vi "Target.vi"() -> ()   [LabVIEW 2019]
uses:
  <vilib>/Platform/TimedLoop/XDataNode/timing_clust.ctl
  <vilib>/Platform/TimedLoop/XDataNode/nitl_modes.ctl
  <vilib>/Platform/TimedLoop/XDataNode/wakeup.ctl
  <vilib>/rvi/Emulation/niFpgaSctlEmulationGetInTimedLoop.vi
  <vilib>/rvi/Emulation/niFpgaEmulationReportErrorSimple.vi
  <vilib>/rvi/Emulation/niFpgaGetClockAttributes.vi
  <vilib>/rvi/Emulation/niFpgaCriticalErrorInLSC.vi
  <vilib>/rvi/DataTransferAndStorage/Container/Common/niFpgaContainerExecOnDevCompGetState.vi
  <vilib>/rvi/errors/niFpgaSetErrorForExecOnDevCompSimple.vi
  <vilib>/rvi/eio/common/nirviEmuReportErrorAndStop.vi
  <vilib>/rvi/interface/RandomDataEmulation/nirviRandomDataAcquireLock.vi
  <vilib>/rvi/interface/RandomDataEmulation/nirviRandomDataQueueStore.vi
  <vilib>/rvi/interface/RandomDataEmulation/nirviRandomDataReleaseLock.vi
  <vilib>/rvi/interface/RandomDataEmulation/nirviFPGAContextMergeError.vi
  <vilib>/rvi/interface/RandomDataEmulation/nirviRandomDataCheckExitLoopConditions.vi
  <vilib>/express/rvi/timingcommon/nirviCommon.vi
  <vilib>/rvi/interface/RandomDataEmulation/niFpgaRandomDataHandleErrors.vi
  <vilib>/rvi/Emulation/niFpgaEmulationIsFPGAContextNoSignature.vi
  <vilib>/rvi/DataTransferAndStorage/Container/Common/niFpgaContainerGetUniqueNameForEmu.vi
  <vilib>/rvi/FIFO/Fifo_Resource/nirvififoEmulationSetSize.vi
  <vilib>/rvi/FIFO/Fifo_Resource/nirviFifoEmulationQueueMgr.vi
  <instcachedir>/0/nirviFifoEmulationQueueMgr_E5CAEC123FF24DC58D834DCA3CDAA9B5.lvgen/nirviFifoEmulationQueueMgr_E5CAEC123FF24DC58D834DCA3CDAA9B5_005.vi
  <vilib>/rvi/FIFO/Fifo_Resource/nirvififoEmulationDetermineInputValidOut.vi
  <vilib>/rvi/FIFO/Fifo_Resource/nirvififoEmulationCreateLock.vi
  <vilib>/rvi/Emulation/niFpgaProcessEmulError.vi
  <vilib>/rvi/FIFO/Fifo_Resource/nirvififoEmulationObtainLock.vi
  <vilib>/rvi/FIFO/Fifo_Resource/nirvififoEmulationReleaseLock.vi
  <vilib>/rvi/occurrence/nirviWaitOnOccurrenceBase.vi
  <vilib>/rvi/errors/nirviReportUnexpectedCaseInternalError.vi
  <vilib>/rvi/errors/nirviReportUnexpectedCaseInternalError (U32).vi
  <vilib>/Utility/error.llb/Clear Errors.vi
  <vilib>/platform/TimedLoop/XDataNode/XDataNode.xnode
  <vilib>/rvi/DataTransferAndStorage/Container/XNode/niFpgaContainer.xnode
  <vilib>/rvi/FIFO/Fifo_Resource/niFpgaFifoEmulationRefInMultiElement.vi
  <vilib>/rvi/FIFO/Fifo_Resource/niFpgaFifoEmulationRefIn.vi
  <vilib>/Platform/TimedLoop/XDataNode/XDNodeRunTimeDep.lvlib
panel:
  out "T3 us":u32 caption="Tick Count(mSec)"
  out "T5 us":u32 caption="Tick Count(mSec)"
  out "T1 us":u32 caption="Tick Count(mSec)"
  out "T5":u32 caption="Tick Count(mSec)"
  out "T4":u32 caption="Tick Count(mSec)"
  out "T3":u32 caption="Tick Count(mSec)"
  out "T2":u32 caption="Tick Count(mSec)"
  out "T1":u32 caption="Tick Count(mSec)"
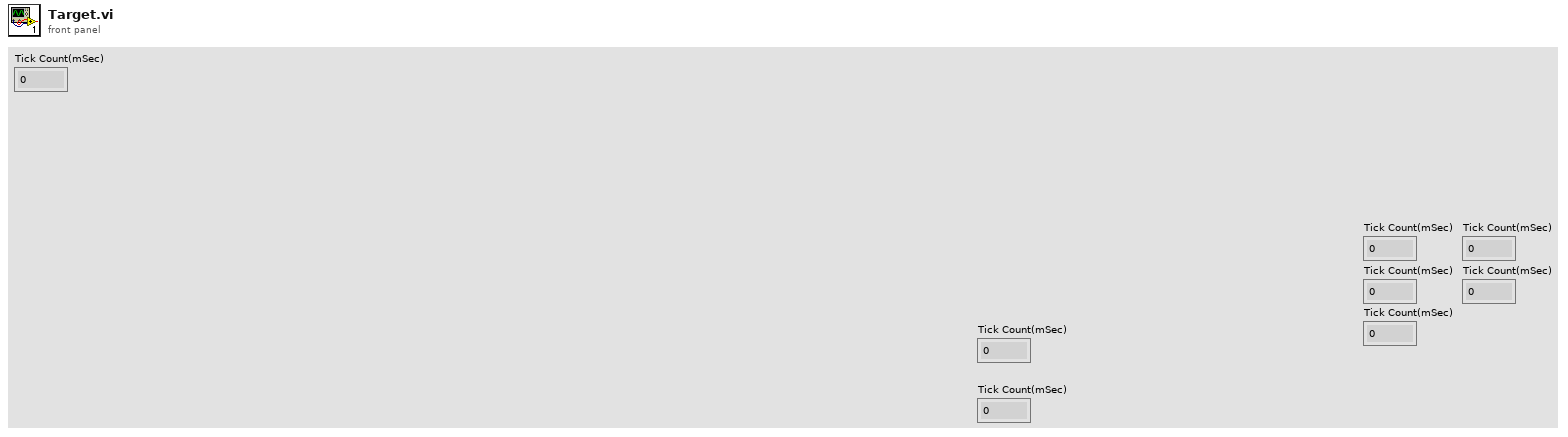
[diagram p1: front panel]
types:
  T1 = typedef "XDNodeRunTimeDep.lvlib/timing_clust.ctl" = cluster{"Expected End [f-1]":u64, "Actual End [f-1]":u64, "Finished Late? [f-1]":bool, "Expected End [i-1]":u64, "Actual End [i-1]":u64, "Finished Late? [i-1]":bool, "Expected Start [i]":u64, "Actual Start [i]":u64, "Expected Start [f]":u64, "Actual Start [f]":u64, "Source Name":string, "Structure Name":string, "Period":i64, "Deadline":i64, "Offset":i64, "Start":i64, "Priority":i32, "Timeout":i32, "Mode":T2, "Wakeup Reason":T3, "Error":errorcluster, "Source Type":string, "Secondary Source Type":string, "Global End Time":u64, "Global Start Time":u64, "Frame Duration":u64, "Iteration Duration":u64, "Assigned CPU":i32, "I/O Scan Engine Mode":u32}
  T2 = typedef "XDNodeRunTimeDep.lvlib/nitl_modes.ctl" = enum32{"No Change", "Process missed periods, maintain original phase", "Discard missed periods, maintain original phase", "Process missed periods, ignore original phase", "Discard missed periods, ignore original phase"}
  T3 = typedef "XDNodeRunTimeDep.lvlib/wakeup.ctl" = enum32{"Normal", "Aborted", "Asynchronous wakeup", "Timing source error", "Timed loop error", "Timeout"}
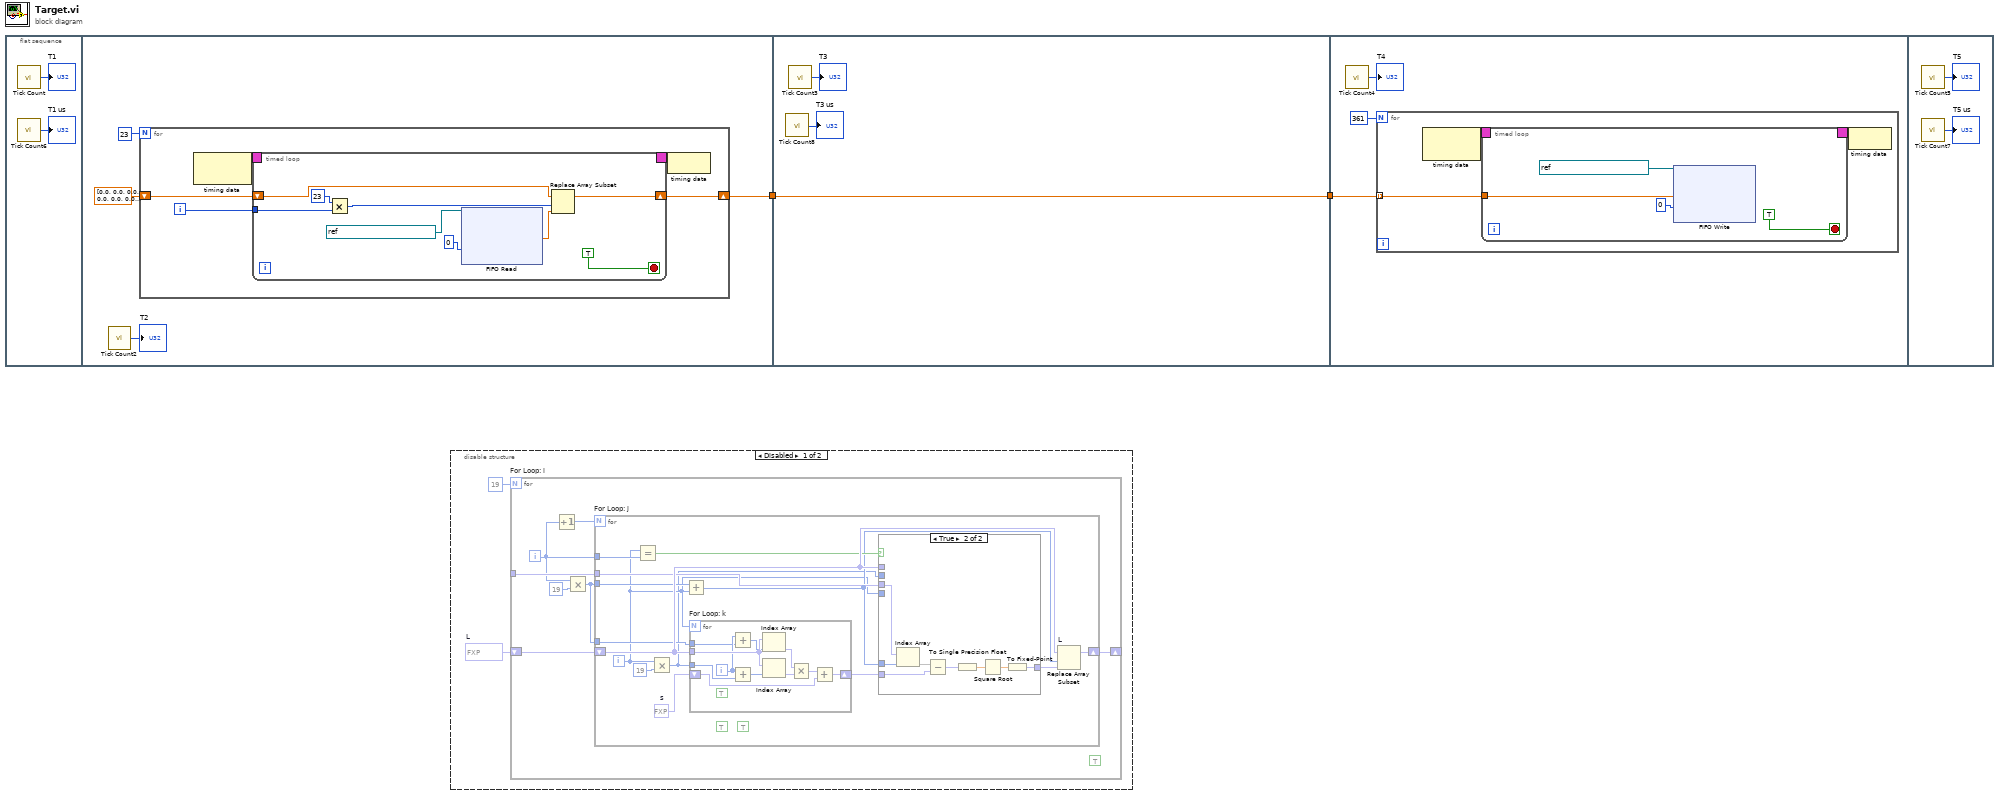
[diagram p0: block diagram]
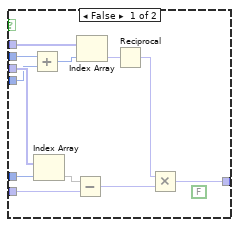
[diagram p2: hidden frame]
diagram:
  n1 = flat-sequence {
    tunnel: [w5] -> w2
    tunnel: w2 -> [w28]
    tunnel: [w28] -> w1
    tunnel: w1 -> [w30]
    frame #0 {
      n2 = call "Tick Count"() -> ("Tick Count(Ticks)"=→"T1":u32)
      n3 = call "Tick Count6"() -> ("Tick Count(uSec)"=→"T1 us":u32)
    }
    frame #1 {
      n4 = call "Tick Count2"() -> ("Tick Count(Ticks)"=→"T2":u32)
      n5 = for {
        N: 23 -> [_]
        shift-right: [w12] -> w5
        shift-left: sgl[] [0.0, 0.0, 0.0, 0.0, 0.0, 0.0, 0.0, 0.0, 0.0, 0.0, 0.0, 0.0, 0.0, 0.0, 0.0, 0.0, 0.0, 0.0, 0.0, 0.0, 0.0, 0.0, 0.0, 0.0, 0.0, 0.0, 0.0, 0.0, 0.0, 0.0, 0.0, 0.0, 0.0, 0.0, 0.0, 0.0, 0.0, 0.0, 0.0, 0.0, 0.0, 0.0, 0.0, 0.0, 0.0, 0.0, 0.0, 0.0, 0.0, 0.0, 0.0, 0.0, 0.0, 0.0, 0.0, 0.0, 0.0, 0.0, 0.0, 0.0, 0.0, 0.0, 0.0, 0.0, 0.0, 0.0, 0.0, 0.0, 0.0, 0.0, 0.0, 0.0, 0.0, 0.0, 0.0, 0.0, 0.0, 0.0, 0.0, 0.0, 0.0, 0.0, 0.0, 0.0, 0.0, 0.0, 0.0, 0.0, 0.0, 0.0, 0.0, 0.0, 0.0, 0.0, 0.0, 0.0, 0.0, 0.0, 0.0, 0.0, 0.0, 0.0, 0.0, 0.0, 0.0, 0.0, 0.0, 0.0, 0.0, 0.0, 0.0, 0.0, 0.0, 0.0, 0.0, 0.0, 0.0, 0.0, 0.0, 0.0, 0.0, 0.0, 0.0, 0.0, 0.0, 0.0, 0.0, 0.0, 0.0, 0.0, 0.0, 0.0, 0.0, 0.0, 0.0, 0.0, 0.0, 0.0, 0.0, 0.0, 0.0, 0.0, 0.0, 0.0, 0.0, 0.0, 0.0, 0.0, 0.0, 0.0, 0.0, 0.0, 0.0, 0.0, 0.0, 0.0, 0.0, 0.0, 0.0, 0.0, 0.0, 0.0, 0.0, 0.0, 0.0, 0.0, 0.0, 0.0, 0.0, 0.0, 0.0, 0.0, 0.0, 0.0, 0.0, 0.0, 0.0, 0.0, 0.0, 0.0, 0.0, 0.0, 0.0, 0.0, 0.0, 0.0, 0.0, 0.0, 0.0, 0.0, 0.0, 0.0, 0.0, 0.0, 0.0, 0.0, 0.0, 0.0, 0.0, 0.0, 0.0, 0.0, 0.0, 0.0, 0.0, 0.0, 0.0, 0.0, 0.0, 0.0, 0.0, 0.0, 0.0, 0.0, 0.0, 0.0, 0.0, 0.0, 0.0, 0.0, 0.0, 0.0, 0.0, 0.0, 0.0, 0.0, 0.0, 0.0, 0.0, 0.0, 0.0, 0.0, 0.0, 0.0, 0.0, 0.0, 0.0, 0.0, 0.0, 0.0, 0.0, 0.0, 0.0, 0.0, 0.0, 0.0, 0.0, 0.0, 0.0, 0.0, 0.0, 0.0, 0.0, 0.0, 0.0, 0.0, 0.0, 0.0, 0.0, 0.0, 0.0, 0.0, 0.0, 0.0, 0.0, 0.0, 0.0, 0.0, 0.0, 0.0, 0.0, 0.0, 0.0, 0.0, 0.0, 0.0, 0.0, 0.0, 0.0, 0.0, 0.0, 0.0, 0.0, 0.0, 0.0, 0.0, 0.0, 0.0, 0.0, 0.0, 0.0, 0.0, 0.0, 0.0, 0.0, 0.0, 0.0, 0.0, 0.0, 0.0, 0.0, 0.0, 0.0, 0.0, 0.0, 0.0, 0.0, 0.0, 0.0, 0.0, 0.0, 0.0, 0.0, 0.0, 0.0, 0.0, 0.0, 0.0, 0.0, 0.0, 0.0, 0.0, 0.0, 0.0, 0.0, 0.0, 0.0, 0.0, 0.0, 0.0, 0.0, 0.0, 0.0, 0.0, 0.0, 0.0, 0.0, 0.0, 0.0, 0.0, 0.0, 0.0, 0.0, 0.0, 0.0, 0.0, 0.0, 0.0, 0.0, 0.0, 0.0, 0.0, 0.0, 0.0, 0.0, 0.0, 0.0, 0.0, 0.0, 0.0, 0.0, 0.0, 0.0, 0.0, 0.0, 0.0, 0.0, 0.0] -> [w13]
        i -> [w11]
        n6 = node-c288() -> (w10:T1)  [unwired: 1 in]
        n7 = timed-loop {
          timing: w10 -> [_]
          timing-out: [_] -> w9
          tunnel: w11 -> [w20]
          shift-right: [w21] -> w12
          shift-left: w13 -> [w22]
          stop <- TRUE stop-if-true
          n8 = Multiply(x=23, y=w20) -> (x*y=w18:i32)
          n9 = xnode ("FIFO Read")("Timeout"=0, "FIFO In"=refnum<k21> "FIFO-host-to-Cholesky") -> ("Element"=w15:sgl[])  [unwired: 2 out]
          n10 = Replace Array Subset(array=w22, new element=w15, index=w18) -> (w21:sgl[])
        }
        n11 = node-c288(w9) -> ()
      }
    }
    frame #2 {
      n12 = call "Tick Count8"() -> ("Tick Count(uSec)"=→"T3 us":u32)
      n13 = call "Tick Count3"() -> ("Tick Count(Ticks)"=→"T3":u32)
    }
    frame #3 {
      n14 = call "Tick Count4"() -> ("Tick Count(Ticks)"=→"T4":u32)
      n15 = for {
        N: 361 -> [_]
        tunnel: w30 -> [w35] mode=indexing
        n16 = node-c288() -> (w34:T1)  [unwired: 1 in]
        n17 = timed-loop {
          tunnel: w35 -> [w38]
          timing: w34 -> [_]
          timing-out: [_] -> w33
          stop <- TRUE stop-if-true
          n18 = xnode ("FIFO Write")("Element"=w38, "Timeout"=0, "FIFO In"=refnum<k21> "FIFO-Cholesky-to-host") -> ()  [unwired: 2 out]
        }
        n19 = node-c288(w33) -> ()
      }
    }
    frame #4 {
      n20 = call "Tick Count5"() -> ("Tick Count(Ticks)"=→"T5":u32)
      n21 = call "Tick Count7"() -> ("Tick Count(mSec)"=→"T5 us":u32)
    }
  }
  n22 = disable-structure shown="Disabled" {
    frame Disabled {
      w47 = fxp<+,1,1>[] [0.0, 0.0, 0.0, 0.0, 0.0, 0.0, 0.0, 0.0, 0.0, 0.0, 0.0, 0.0, 0.0, 0.0, 0.0, 0.0, 0.0, 0.0, 0.0, 0.0, 0.0, 0.0, 0.0, 0.0, 0.0, 0.0, 0.0, 0.0, 0.0, 0.0, 0.0, 0.0, 0.0, 0.0, 0.0, 0.0, 0.0, 0.0, 0.0, 0.0, 0.0, 0.0, 0.0, 0.0, 0.0, 0.0, 0.0, 0.0, 0.0, 0.0, 0.0, 0.0, 0.0, 0.0, 0.0, 0.0, 0.0, 0.0, 0.0, 0.0, 0.0, 0.0, 0.0, 0.0, 0.0, 0.0, 0.0, 0.0, 0.0, 0.0, 0.0, 0.0, 0.0, 0.0, 0.0, 0.0, 0.0, 0.0, 0.0, 0.0, 0.0, 0.0, 0.0, 0.0, 0.0, 0.0, 0.0, 0.0, 0.0, 0.0, 0.0, 0.0, 0.0, 0.0, 0.0, 0.0, 0.0, 0.0, 0.0, 0.0, 0.0, 0.0, 0.0, 0.0, 0.0, 0.0, 0.0, 0.0, 0.0, 0.0, 0.0, 0.0, 0.0, 0.0, 0.0, 0.0, 0.0, 0.0, 0.0, 0.0, 0.0, 0.0, 0.0, 0.0, 0.0, 0.0, 0.0, 0.0, 0.0, 0.0, 0.0, 0.0, 0.0, 0.0, 0.0, 0.0, 0.0, 0.0, 0.0, 0.0, 0.0, 0.0, 0.0, 0.0, 0.0, 0.0, 0.0, 0.0, 0.0, 0.0, 0.0, 0.0, 0.0, 0.0, 0.0, 0.0, 0.0, 0.0, 0.0, 0.0, 0.0, 0.0, 0.0, 0.0, 0.0, 0.0, 0.0, 0.0, 0.0, 0.0, 0.0, 0.0, 0.0, 0.0, 0.0, 0.0, 0.0, 0.0, 0.0, 0.0, 0.0, 0.0, 0.0, 0.0, 0.0, 0.0, 0.0, 0.0, 0.0, 0.0, 0.0, 0.0, 0.0, 0.0, 0.0, 0.0, 0.0, 0.0, 0.0, 0.0, 0.0, 0.0, 0.0, 0.0, 0.0, 0.0, 0.0, 0.0, 0.0, 0.0, 0.0, 0.0, 0.0, 0.0, 0.0, 0.0, 0.0, 0.0, 0.0, 0.0, 0.0, 0.0, 0.0, 0.0, 0.0, 0.0, 0.0, 0.0, 0.0, 0.0, 0.0, 0.0, 0.0, 0.0, 0.0, 0.0, 0.0, 0.0, 0.0, 0.0, 0.0, 0.0, 0.0, 0.0, 0.0, 0.0, 0.0, 0.0, 0.0, 0.0, 0.0, 0.0, 0.0, 0.0, 0.0, 0.0, 0.0, 0.0, 0.0, 0.0, 0.0, 0.0, 0.0, 0.0, 0.0, 0.0, 0.0, 0.0, 0.0, 0.0, 0.0, 0.0, 0.0, 0.0, 0.0, 0.0, 0.0, 0.0, 0.0, 0.0, 0.0, 0.0, 0.0, 0.0, 0.0, 0.0, 0.0, 0.0, 0.0, 0.0, 0.0, 0.0, 0.0, 0.0, 0.0, 0.0, 0.0, 0.0, 0.0, 0.0, 0.0, 0.0, 0.0, 0.0, 0.0, 0.0, 0.0, 0.0, 0.0, 0.0, 0.0, 0.0, 0.0, 0.0, 0.0, 0.0, 0.0, 0.0, 0.0, 0.0, 0.0, 0.0, 0.0, 0.0, 0.0, 0.0, 0.0, 0.0, 0.0, 0.0, 0.0, 0.0, 0.0, 0.0, 0.0, 0.0, 0.0, 0.0, 0.0, 0.0, 0.0, 0.0, 0.0, 0.0, 0.0, 0.0, 0.0, 0.0, 0.0, 0.0, 0.0, 0.0, 0.0, 0.0, 0.0, 0.0, 0.0, 0.0, 0.0, 0.0, 0.0]  # L
      n23 = for "For Loop: i" {
        N: 19 -> [_]
        shift-right: [w53] -> _
        shift-left: w47 -> [w55]
        tunnel: [w52] -> w48
        i -> [w51]
        (unwired) TRUE
        n24 = Increment(x=w51) -> (x+1=w54:i32)
        n25 = Multiply(x=w51, y=19) -> (x*y=w50:i32)
        n26 = for "For Loop: j" {
          N: w54 -> [_]
          tunnel: w51 -> [w65]
          shift-right: [w67] -> w53
          shift-left: w55 -> [w66]
          tunnel: w52 -> [w64]
          tunnel: w50 -> [w61]
          tunnel: w50 -> [w60]
          i -> [w59]
          (unwired) TRUE
          (unwired) TRUE
          w69 = fxp<+,1,1> 0.0  # s
          n27 = Equal?(x=w59, y=w65) -> (x = y?=w63:bool)
          n28 = Multiply(x=w59, y=19) -> (x*y=w58:i32)
          n29 = Add(x=w61, y=w59) -> (x+y=w62:i32)
          n30 = for "For Loop: k" {
            N: w59 -> [_]
            tunnel: w66 -> [w100]
            shift-right: [w98] -> w68
            shift-left: w69 -> [w99]
            tunnel: w60 -> [w96]
            tunnel: w58 -> [w95]
            i -> [w97]
            (unwired) TRUE
            n31 = Add(x=w97, y=w96) -> (x+y=w91:i32)
            n32 = Add(x=w97, y=w95) -> (x+y=w90:i32)
            n33 = Index Array(array=w100, index=w91) -> (element=w94:fxp<+,1,1>)
            n34 = Index Array(array=w100, index=w90) -> (element=w93:fxp<+,1,1>)
            n35 = Multiply(x=w94, y=w93) -> (x*y=w92:fxp<+,1,1>)
            n36 = Add(x=w92, y=w99) -> (x+y=w98:fxp<+,1,1>)
          }
          n37 = case shown="True" w63 {
            tunnel: w68 -> [w73 w89]
            tunnel: w66 -> [w81 _]
            tunnel: w64 -> [w78 w88]
            tunnel: w62 -> [w77 w87]
            tunnel: w59 -> [w76 _]
            tunnel: w58 -> [w75 _]
            tunnel: [w74 w86] -> w57
            frame False {
              (unwired) FALSE
              n38 = Add(x=w75, y=w76) -> (x+y=w71:i32)
              n39 = Index Array(array=w78, index=w77) -> (element=w70)
              n40 = Subtract(x=w70, y=w73) -> (x-y=w72:fxp<+,1,1>)
              n41 = Index Array(array=w81, index=w71) -> (element=w80:fxp<+,1,1>)
              n42 = Reciprocal(x=w80) -> (1/x=w79:fxp<+,2,1>)
              n43 = Multiply(x=w79, y=w72) -> (x*y=w74:fxp<+,1,0>)
            }
            frame True {
              n44 = Index Array(array=w88, index=w87) -> (element=w82)
              n45 = Subtract(x=w82, y=w89) -> (x-y=w84:fxp<+,1,1>)
              n46 = To Single Precision Float(number=w84) -> (single precision float=w83:sgl)
              n47 = Square Root(x=w83) -> (sqrt(x)=w85:sgl)
              n48 = To Fixed-Point(number=w85) -> (fixed-point=w86:fxp<+/-,32,16>)  [unwired: 1 in]
            }
          }
          n49 = Replace Array Subset "L"(array=w66, new element=w57, index=w62) -> (w67:fxp<+,1,1>[])
        }
      }
    }
    frame Enabled {
    }
  }
